vi "Resize Window.vi"(8 "error in (no error)":errorcluster, 9 "new size (100,100)":cluster{"width":i16, "height":i16}={"width"=100, "height"=100}, 10 "window name (\"\")":string, 11 "window refnum (NaWR)":T1) -> (0 "error out":errorcluster, 1 "prev size":cluster{"width":i16, "height":i16}, 3 "window refnum out":T1)   [LabVIEW 2020, in "MacroAssert.lvlib" / "WINUTIL.lvlib"]
doc: "This function will resize (without moving) the window named in the window name input or identified by the window refnum. Window size is determined in pixels. If the window cannot be found, an error will be returned."
uses:
  WINUTIL.lvlib
  Window Refnum.ctl
  user32.dll
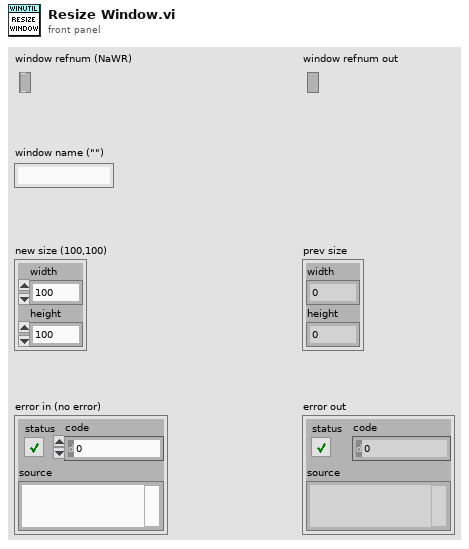
[diagram p1: front panel]
types:
  T1 = typedef "MacroAssert.lvlib/WINUTIL.lvlib/Window Refnum.ctl" = refnum<k1>
  T2 = typedef "MacroAssert.lvlib/WINUTIL.lvlib/Window Rectangle.ctl" = cluster{"left":i16, "top":i16, "right":i16, "bottom":i16}
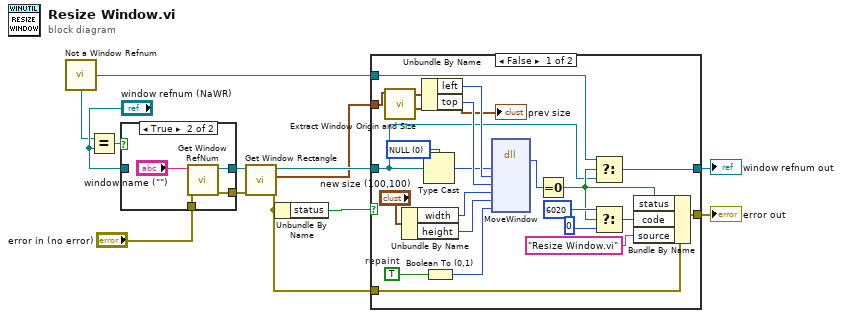
[diagram p0: block diagram]
diagram:
  n1 = call "Not a Window Refnum.vi"() -> ("Not a Window Refnum"=w2:T1)
  n2 = Equal?(x=w2, y="window refnum (NaWR)") -> (x = y?=w4:bool)
  n3 = case shown="True" w4 {
    tunnel: "error in (no error)" -> [w14 w18]
    tunnel: [w14 w16] -> w11
    tunnel: [w13 w17] -> w10
    tunnel: "window refnum (NaWR)" -> [w13 _]
    frame False {
    }
    frame True {
      n4 = call "Get Window RefNum.vi"("error in (no error)"=w18, "window name (\"\")"="window name (\"\")") -> ("error out"=w16:errorcluster, "window refnum (NaWR)"=w17:T1)  [unwired: 8 in]
    }
  }
  n5 = call "Get Window Rectangle.vi"("error in (no error)"=w11, "window refnum (NaWR)"=w10) -> ("error out"=w5:errorcluster, "window rect"=w7:T2, "window refnum out"=w8:T1)  [unwired: 7 in]
  n6 = Unbundle By Name(w5) -> ("status"=w6:bool)
  n7 = case shown="False" w6 {
    tunnel: w7 -> [w41 _]
    tunnel: [w32 w43] -> w12
    tunnel: w8 -> [w20 w42]
    tunnel: [w24 w42] -> w1
    tunnel: w5 -> [w25 w43]
    tunnel: w2 -> [w19 _]
    frame False {
      w21 = u32 0 items=["NULL"]
      w39 = TRUE  # repaint
      n8 = call "Extract Window Origin and Size.vi"("window rect"=w41) -> ("window size"=→"prev size":cluster{"width":i16, "height":i16}, "window origin"=w31:cluster{"left":i16, "top":i16})  [unwired: 9 in]
      n9 = Unbundle By Name("new size (100,100)") -> ("width"=w28:i16, "height"=w27:i16)
      n10 = Unbundle By Name(w31) -> ("left"=w30:i16, "top"=w29:i16)
      n11 = Type Cast(type=w21, x=w20) -> (*(type *) &x=w22:u32)
      n12 = Boolean To (0,1)(Boolean=w39) -> (0, 1=w38:i16)
      n13 = dll-call lib="USER32.DLL" fn="MoveWindow"("hWnd"=w22, "left"=w30, "top"=w29, "right"=w28, "bottom"=w27, "repaint"=w38) -> ("error"=w37:i32)  [unwired: 4 in, 7 out]
      n14 = Equal To 0?(x=w37) -> (x = 0?=w23:bool)
      n15 = Select(t=w19, s=w23, f=w20) -> (s? t:f=w24:T1)
      n16 = Select(t=6020, s=w23, f=0) -> (s? t:f=w33:i32)
      n17 = Bundle By Name(cluster=w25, "status"=w23, "code"=w33, "source"="Resize Window.vi") -> (w32:errorcluster)
    }
    frame True {
    }
  }
  "error out" <- w12
  "window refnum out" <- w1
